vi "Facade.vi"(0 "Data In":T9, 2 "Display State In":T4={"Z_Source"={"connect"=FALSE, "Z_Source"=enum."initialize", "Z_State_heating"=enum."on"}, "Write"=FALSE, "Z1_ind"=0, "button state"=enum."init", "reset_timer"=FALSE, "load_timer"=FALSE, "end_timer"=TRUE}, 3 "Container State":T8) -> (6 "Data Out":T9, 7 "Display State Out":T4={"Z_Source"={"connect"=FALSE, "Z_Source"=enum."initialize", "Z_State_heating"=enum."on"}, "Write"=FALSE, "Z1_ind"=0, "button state"=enum."init", "reset_timer"=FALSE, "load_timer"=FALSE, "end_timer"=TRUE}, 8 "Action":T3)   [LabVIEW 2019, in "Heating.lvlib" / "Z_OnSwitch.xctl"]
uses:
  Z_OnSwitch.xctl
  Data.ctl
  <vilib>/_xctls/Container State.ctl
  State.ctl
  Z_source.ctl
  Z_State.ctl
  On_ButtonState.ctl
  <vilib>/_xctls/Action.ctl
  Z_OnSwitch.ctl
  Z_OnInd.ctl
  <vilib>/_xctls/XControlSupport.lvlib
  Timer Delay/Timers.lvlib
  Heating.lvlib
panel:
  in  "Z_OnSwitch":T1
  out "Z1 ind":T2
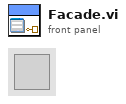
[diagram p1: front panel]
types:
  T1 = typedef "Heating.lvlib/Z_OnSwitch.xctl/Z_OnSwitch.ctl" = bool
  T2 = typedef "Heating.lvlib/Z_OnSwitch.xctl/Z_OnInd.ctl" = u8
  T3 = typedef "XControlSupport.lvlib/Action.ctl" = cluster{"Data Changed?":bool, "State Changed?":bool, "Action Name":string}
  T4 = typedef "Heating.lvlib/Z_OnSwitch.xctl/State.ctl" = cluster{"Z_Source":cluster{"connect":bool, "Z_Source":T5, "Z_State_heating":T6}, "Write":bool, "Z1_ind":u8, "button state":T7, "reset_timer":bool, "load_timer":bool, "end_timer":bool}
  T5 = typedef "Heating.lvlib/Z_source.ctl" = enum8{"initialize", "local disabled", "local hand", "hand", "auto", "dist"}
  T6 = typedef "Heating.lvlib/Z_State.ctl" = enum8{"initialization", "alarm", "disabled", "not ready", "stop ready", "reserv", "switched off", "reserv2", "switched on", "check", "on min", "decrease out", "on", "increase out", "on max"}
  T7 = typedef "Heating.lvlib/Z_OnSwitch.xctl/On_ButtonState.ctl" = enum16{"init", "not connect", "local disabled", "local hand", "switch off", "off", "switch on", "on", "auto", "dist"}
  T8 = typedef "XControlSupport.lvlib/Container State.ctl" = cluster{"Indicator?":bool, "Run Mode?":bool, " Refnum":refnum<vi>}
  T9 = typedef "Heating.lvlib/Z_OnSwitch.xctl/Data.ctl" = bool
  T10 = enum8{"Enabled", "Disabled", "Disabled and Grayed Out"}
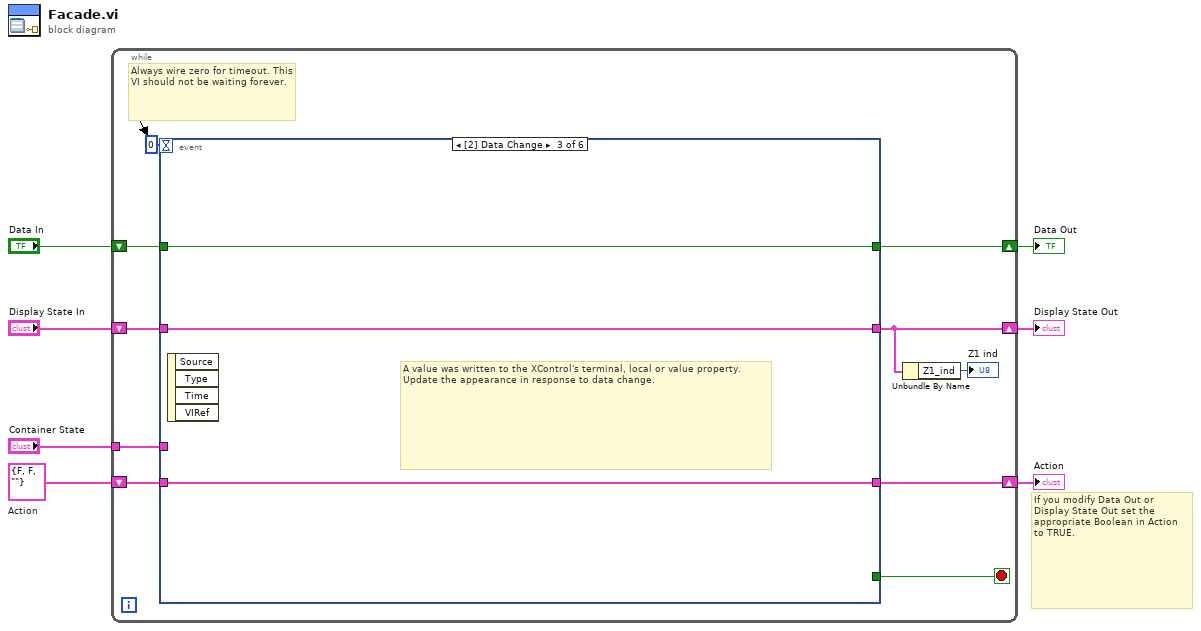
[diagram p0: block diagram]
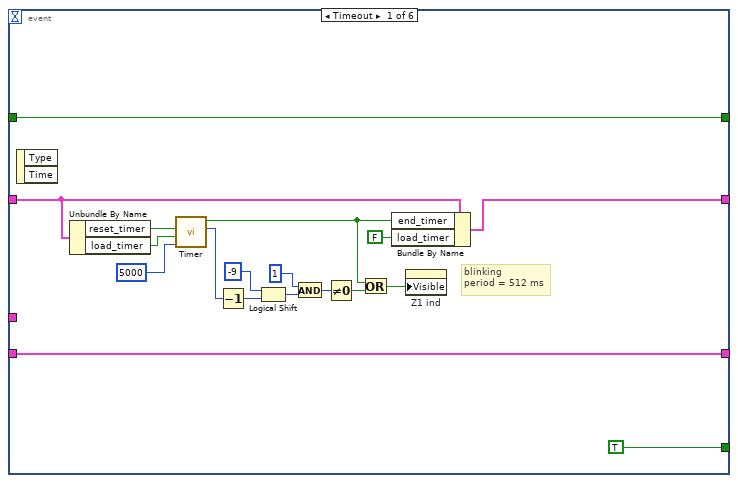
[diagram p2: hidden frame]
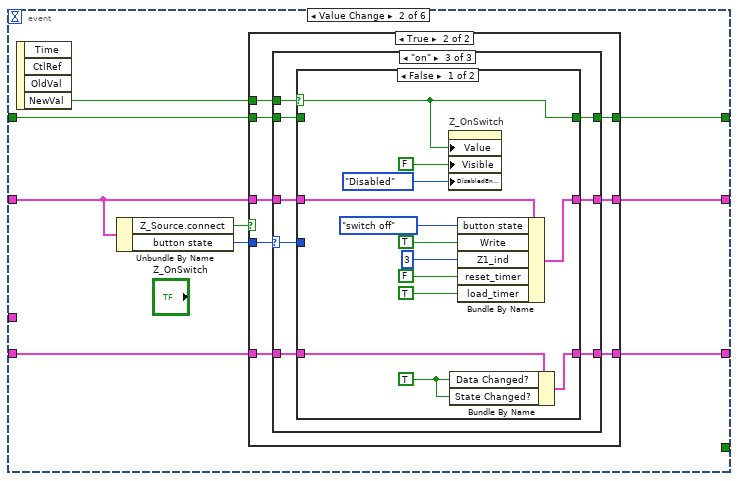
[diagram p3: hidden frame]
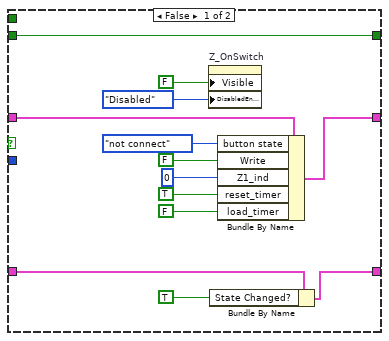
[diagram p4: hidden frame]
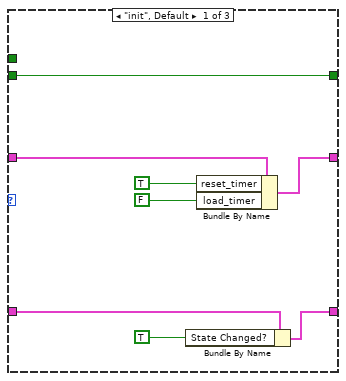
[diagram p5: hidden frame]
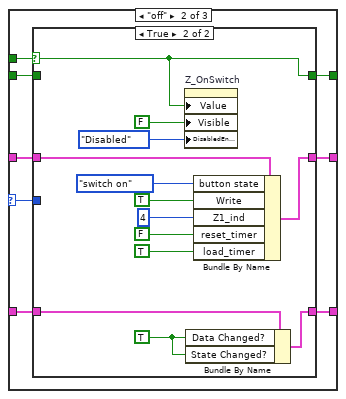
[diagram p6: hidden frame]
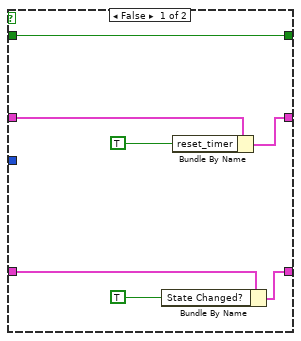
[diagram p7: hidden frame]
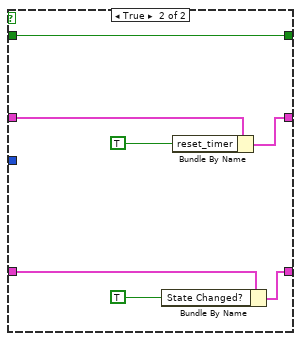
[diagram p8: hidden frame]
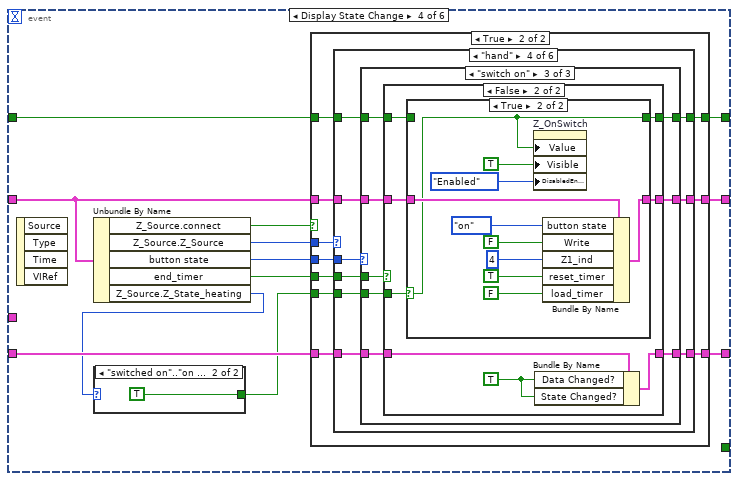
[diagram p9: hidden frame]
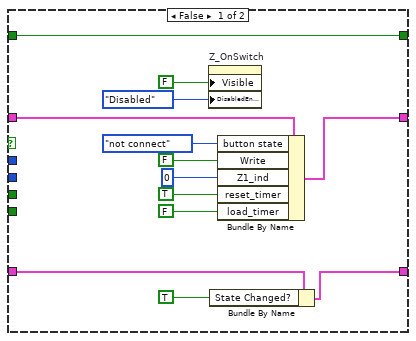
[diagram p11: hidden frame]
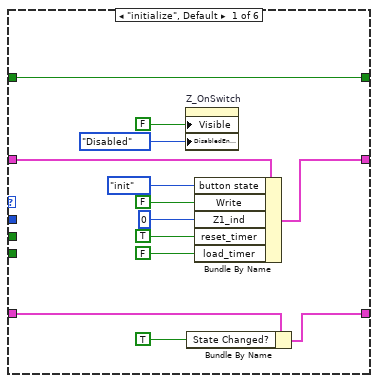
[diagram p12: hidden frame]
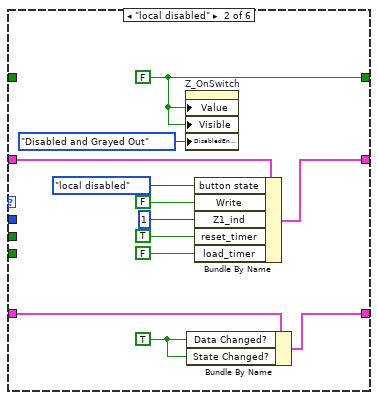
[diagram p13: hidden frame]
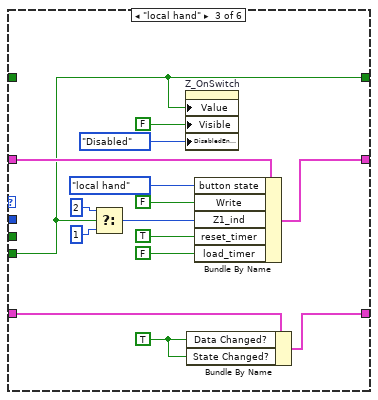
[diagram p14: hidden frame]
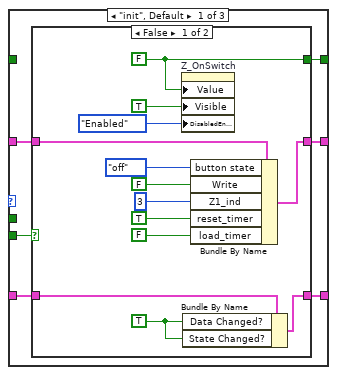
[diagram p15: hidden frame]
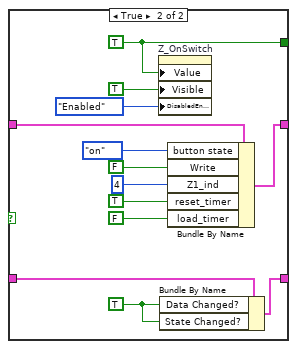
[diagram p16: hidden frame]
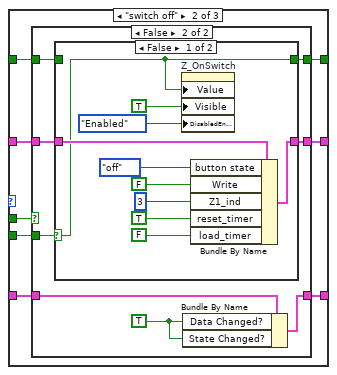
[diagram p17: hidden frame]
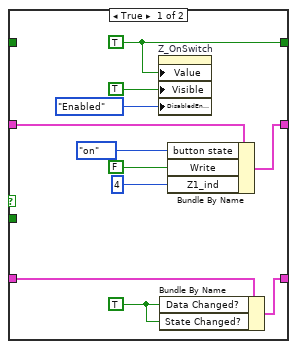
[diagram p18: hidden frame]
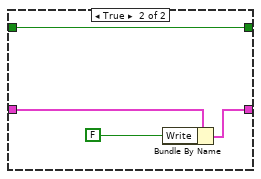
[diagram p19: hidden frame]
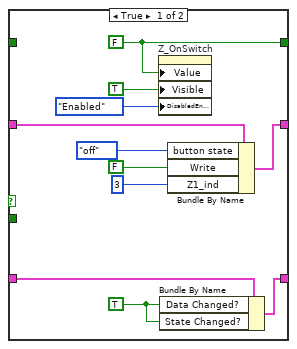
[diagram p20: hidden frame]
diagram:
  w1 = T3 {"Data Changed?"=FALSE, "State Changed?"=FALSE, "Action Name"=""}  # Action
  # "If you modify Data Out or\nDisplay State Out set the\nappropriate Boolean in Action\nto TRUE."
  n1 = while {
    shift-right: [w8] -> w4
    shift-left: "Display State In" -> [w17]
    tunnel: "Container State" -> [w14]
    shift-right: [w12] -> w7
    shift-left: "Data In" -> [w13]
    shift-right: [w10] -> w2
    shift-left: w1 -> [w11]
    stop <- w16 stop-if-true
    # "Always wire zero for timeout. This\nVI should not be waiting forever."
    n2 = event shown="[2] Data Change" {
      selector: _ -> [_ _ _ _ _ _]
      dyn-events: _ -> [_ _ _ _ _ _]
      timeout: 0 -> [_ _ _ _ _ _]
      tunnel: w17 -> [w30 w38 w131 w138 w362 w366]
      tunnel: [w29 w43 w131 w142 w362 w366] -> w8
      tunnel: [TRUE _ _ _ _ _] -> w16
      tunnel: w14 -> [_ _ _ _ w363 w367]
      tunnel: w13 -> [w33 w42 w132 w144 w361 w365]
      tunnel: [w33 w41 w132 w143 w361 w365] -> w12
      tunnel: [w34 w39 w130 w140 w360 w364] -> w10
      tunnel: w11 -> [w34 w40 w130 w141 w360 w364]
      event Timeout {
        # "blinking\nperiod = 512 ms"
        n3 = event-data() -> ()  [unwired: 1 in, 2 out]
        n4 = Unbundle By Name(w30) -> ("reset_timer"=w32:bool, "load_timer"=w31:bool)
        n5 = call "Timer.vi"("ms"=5000, "Load (F)"=w31, "Reset (F)"=w32) -> ("t ms"=w27:u32, "End"=w23:bool)  [unwired: 6 in]
        n6 = Decrement(x=w27) -> (x-1=w22:u32)
        n7 = Logical Shift(y=i16 -9, x=w22) -> (x << y=w20:u32)
        n8 = And(x=u32 1 ("y"), y=w20) -> (x .and. y?=w18:u32)
        n9 = Not Equal To 0?(x=w18) -> (x != 0?=w24:bool)
        n10 = Or(x=w23, y=w24) -> (x .or. y?=w25:bool)
        n11 = Bundle By Name(cluster=w30, "end_timer"=w23, "load_timer"=FALSE) -> (w29:T4)
        n12 = property on="Z1 ind" class="Ring (strict)"("Visible"=w25) -> ()  [unwired: 2 in, 2 out]
      }
      event Value Change {
        n13 = event-data() -> ("NewVal"=w44:T1)  [unwired: 1 in, 3 out]
        n14 = Unbundle By Name(w38) -> ("Z_Source.connect"=w37:bool, "button state"=w36:T7)
        n15 = case shown="True" w37 {
          tunnel: w36 -> [_ w65]
          tunnel: w44 -> [_ w64]
          tunnel: w38 -> [w52 w63]
          tunnel: [w51 w62] -> w43
          tunnel: w42 -> [w57 w61]
          tunnel: [w57 w60] -> w41
          tunnel: w40 -> [w49 w58]
          tunnel: [w48 w59] -> w39
          frame False {
            n16 = property on="Z_OnSwitch" class="Bool (strict)"("Visible"=FALSE ("Z_ASwitch"), "DisabledEnum"=T10."Disabled" ("Disabled")) -> ()  [unwired: 2 in, 2 out]
            n17 = Bundle By Name(cluster=w49, "State Changed?"=TRUE ("Data Changed?")) -> (w48:T3)
            n18 = Bundle By Name(cluster=w52, "button state"=On_ButtonState."not connect" ("f 3"), "Write"=FALSE ("Z_ASwitch"), "Z1_ind"=u8 0 ("Z1_ind visu"), "reset_timer"=TRUE ("Z_ASwitch"), "load_timer"=FALSE ("Z_ASwitch")) -> (w51:T4)
          }
          frame True {
            n19 = case shown="\"on\"" w65 {
              selector: w65 -> [_ w80 w108]
              tunnel: w64 -> [_ w81 w109]
              tunnel: w63 -> [w72 w79 w107]
              tunnel: [w71 w78 w106] -> w62
              tunnel: w61 -> [w70 w76 w105]
              tunnel: [w70 w77 w104] -> w60
              tunnel: [w67 w74 w102] -> w59
              tunnel: w58 -> [w68 w75 w103]
              frame "init", Default {
                # "local hand"
                n20 = Bundle By Name(cluster=w68, "State Changed?"=TRUE ("Data Changed?")) -> (w67:T3)
                n21 = Bundle By Name(cluster=w72, "reset_timer"=TRUE, "load_timer"=FALSE) -> (w71:T4)
              }
              frame "off" {
                # "local hand"
                n22 = case shown="True" w81 {
                  selector: w81 -> [_ w93]
                  tunnel: w80 -> [_ _]
                  tunnel: w79 -> [w87 w95]
                  tunnel: [w86 w94] -> w78
                  tunnel: [w85 w93] -> w77
                  tunnel: w76 -> [w85 _]
                  tunnel: w75 -> [w83 w91]
                  tunnel: [w82 w90] -> w74
                  frame False {
                    n23 = Bundle By Name(cluster=w83, "State Changed?"=TRUE ("Data Changed?")) -> (w82:T3)
                    n24 = Bundle By Name(cluster=w87, "reset_timer"=TRUE) -> (w86:T4)
                  }
                  frame True {
                    w92 = TRUE ("Data Changed?")
                    n25 = property on="Z_OnSwitch" class="Bool (strict)"("Value"=w93, "Visible"=FALSE ("Z_ASwitch"), "DisabledEnum"=T10."Disabled" ("Disabled")) -> ()  [unwired: 2 in, 2 out]
                    n26 = Bundle By Name(cluster=w91, "Data Changed?"=w92, "State Changed?"=w92) -> (w90:T3)
                    n27 = Bundle By Name(cluster=w95, "button state"=On_ButtonState."switch on" ("f 3"), "Write"=TRUE ("Z_ASwitch"), "Z1_ind"=u8 4 ("Z1_ind visu"), "reset_timer"=FALSE ("Z_ASwitch"), "load_timer"=TRUE ("Z_ASwitch")) -> (w94:T4)
                  }
                }
              }
              frame "on" {
                # "local hand"
                n28 = case shown="False" w109 {
                  selector: w109 -> [w114 _]
                  tunnel: w108 -> [_ _]
                  tunnel: w107 -> [w116 w128]
                  tunnel: [w115 w127] -> w106
                  tunnel: w105 -> [_ w129]
                  tunnel: [w114 w129] -> w104
                  tunnel: w103 -> [w112 w124]
                  tunnel: [w111 w123] -> w102
                  frame False {
                    w113 = TRUE ("Data Changed?")
                    n29 = property on="Z_OnSwitch" class="Bool (strict)"("Value"=w114, "Visible"=FALSE ("Z_ASwitch"), "DisabledEnum"=T10."Disabled" ("Disabled")) -> ()  [unwired: 2 in, 2 out]
                    n30 = Bundle By Name(cluster=w112, "Data Changed?"=w113, "State Changed?"=w113) -> (w111:T3)
                    n31 = Bundle By Name(cluster=w116, "button state"=On_ButtonState."switch off" ("f 3"), "Write"=TRUE ("Z_ASwitch"), "Z1_ind"=u8 3 ("Z1_ind visu"), "reset_timer"=FALSE ("Z_ASwitch"), "load_timer"=TRUE ("Z_ASwitch")) -> (w115:T4)
                  }
                  frame True {
                    n32 = Bundle By Name(cluster=w124, "State Changed?"=TRUE ("Data Changed?")) -> (w123:T3)
                    n33 = Bundle By Name(cluster=w128, "reset_timer"=TRUE ("Z1_ind_blinking")) -> (w127:T4)
                  }
                }
              }
            }
          }
        }
      }
      event Data Change {
        # "A value was written to the XControl's terminal, local or value property.\nUpdate the appearance in response to data change."
        n34 = event-data() -> ()  [unwired: 1 in, 4 out]
      }
      event Display State Change {
        n35 = event-data() -> ()  [unwired: 1 in, 4 out]
        n36 = Unbundle By Name(w138) -> ("Z_Source.connect"=w139:bool, "Z_Source.Z_Source"=w136:T5, "button state"=w135:T7, "end_timer"=w137:bool, "Z_Source.Z_State_heating"=w134:T6)
        n37 = case shown="\"switched on\"..\"on max\"" w134 {
          tunnel: [_ TRUE] -> w133
          frame "initialization", Default {
          }
          frame "switched on".."on max" {
          }
        }
        n38 = case shown="True" w139 {
          tunnel: w136 -> [_ w168]
          tunnel: w138 -> [w153 w167]
          tunnel: [w152 w166] -> w142
          tunnel: w144 -> [w158 w165]
          tunnel: [w158 w164] -> w143
          tunnel: w141 -> [w150 w162]
          tunnel: [w149 w163] -> w140
          tunnel: w137 -> [_ w161]
          tunnel: w135 -> [_ w160]
          tunnel: w133 -> [_ w159]
          frame False {
            n39 = property on="Z_OnSwitch" class="Bool (strict)"("Visible"=FALSE ("Z_ASwitch"), "DisabledEnum"=T10."Disabled" ("Disabled")) -> ()  [unwired: 2 in, 2 out]
            n40 = Bundle By Name(cluster=w150, "State Changed?"=TRUE ("Data Changed?")) -> (w149:T3)
            n41 = Bundle By Name(cluster=w153, "button state"=On_ButtonState."not connect" ("f 3"), "Write"=FALSE ("Z_ASwitch"), "Z1_ind"=u8 0 ("Z1_ind visu"), "reset_timer"=TRUE ("Z_ASwitch"), "load_timer"=FALSE ("Z_ASwitch")) -> (w152:T4)
          }
          frame True {
            n42 = case shown="\"hand\"" w168 {
              tunnel: w167 -> [w181 w193 w208 w214 w346 w359]
              tunnel: [w180 w192 w207 w216 w345 w358] -> w166
              tunnel: w165 -> [w170 _ _ w215 _ _]
              tunnel: [w170 w183 w194 w217 w332 w347] -> w164
              tunnel: [w178 w190 w205 w210 w343 w356] -> w163
              tunnel: w162 -> [w179 w191 w206 w211 w344 w357]
              tunnel: w161 -> [_ _ _ w213 _ _]
              tunnel: w160 -> [_ _ _ w212 _ _]
              tunnel: w159 -> [_ _ w194 w209 w332 w347]
              frame "initialize", Default {
                # "local hand"
                n43 = property on="Z_OnSwitch" class="Bool (strict)"("Visible"=FALSE ("Z_ASwitch"), "DisabledEnum"=T10."Disabled" ("Disabled")) -> ()  [unwired: 2 in, 2 out]
                n44 = Bundle By Name(cluster=w179, "State Changed?"=TRUE ("Data Changed?")) -> (w178:T3)
                n45 = Bundle By Name(cluster=w181, "button state"=On_ButtonState."init" ("f 3"), "Write"=FALSE ("Z_ASwitch"), "Z1_ind"=u8 0 ("Z1_ind visu"), "reset_timer"=TRUE ("Z_ASwitch"), "load_timer"=FALSE ("Z_ASwitch")) -> (w180:T4)
              }
              frame "local disabled" {
                w182 = TRUE ("Data Changed?")
                w183 = FALSE ("Z_ASwitch")
                # "local hand"
                n46 = property on="Z_OnSwitch" class="Bool (strict)"("Value"=w183, "Visible"=w183, "DisabledEnum"=T10."Disabled and Grayed Out" ("Disabled")) -> ()  [unwired: 2 in, 2 out]
                n47 = Bundle By Name(cluster=w191, "Data Changed?"=w182, "State Changed?"=w182) -> (w190:T3)
                n48 = Bundle By Name(cluster=w193, "button state"=On_ButtonState."local disabled" ("f 3"), "Write"=FALSE ("Z_ASwitch"), "Z1_ind"=u8 1 ("Z1_ind visu"), "reset_timer"=TRUE ("Z_ASwitch"), "load_timer"=FALSE ("Z_ASwitch")) -> (w192:T4)
              }
              frame "local hand" {
                w198 = TRUE ("Data Changed?")
                # "local hand"
                n49 = Select(t=u8 2 ("Z1_ind visu"), s=w194, f=u8 1 ("Z1_ind visu")) -> (s? t:f=w195:u8)
                n50 = property on="Z_OnSwitch" class="Bool (strict)"("Value"=w194, "Visible"=FALSE ("Z_ASwitch"), "DisabledEnum"=T10."Disabled" ("Disabled")) -> ()  [unwired: 2 in, 2 out]
                n51 = Bundle By Name(cluster=w206, "Data Changed?"=w198, "State Changed?"=w198) -> (w205:T3)
                n52 = Bundle By Name(cluster=w208, "button state"=On_ButtonState."local hand" ("f 3"), "Write"=FALSE ("Z_ASwitch"), "Z1_ind"=w195, "reset_timer"=TRUE ("Z_ASwitch"), "load_timer"=FALSE ("Z_ASwitch")) -> (w207:T4)
              }
              frame "hand" {
                # "local hand"
                n53 = case shown="\"switch on\"" w212 {
                  tunnel: w213 -> [_ w257 w298]
                  tunnel: w214 -> [w223 w251 w292]
                  tunnel: [w219 w252 w293] -> w216
                  tunnel: w215 -> [_ w256 w297]
                  tunnel: [w220 w255 w296] -> w217
                  tunnel: w211 -> [w222 w253 w294]
                  tunnel: [w221 w254 w295] -> w210
                  tunnel: w209 -> [w218 w250 w291]
                  frame "init", Default {
                    n54 = case shown="False" w218 {
                      tunnel: w223 -> [w233 w246]
                      tunnel: w222 -> [w231 w244]
                      tunnel: [w230 w243] -> w221
                      tunnel: [w229 w242] -> w220
                      tunnel: [w224 w237] -> w219
                      frame False {
                        w225 = TRUE ("Data Changed?")
                        w229 = FALSE ("Z_ASwitch")
                        n55 = property on="Z_OnSwitch" class="Bool (strict)"("Value"=w229, "Visible"=TRUE ("Z_ASwitch"), "DisabledEnum"=T10."Enabled" ("Disabled")) -> ()  [unwired: 2 in, 2 out]
                        n56 = Bundle By Name(cluster=w231, "Data Changed?"=w225, "State Changed?"=w225) -> (w230:T3)
                        n57 = Bundle By Name(cluster=w233, "button state"=On_ButtonState."off" ("f 3"), "Write"=FALSE ("Z_ASwitch"), "Z1_ind"=u8 3 ("Z1_ind visu"), "reset_timer"=TRUE ("Z_ASwitch"), "load_timer"=FALSE ("Z_ASwitch")) -> (w224:T4)
                      }
                      frame True {
                        w238 = TRUE ("Data Changed?")
                        w242 = TRUE ("Z_ASwitch")
                        n58 = property on="Z_OnSwitch" class="Bool (strict)"("Value"=w242, "Visible"=TRUE ("Z_ASwitch"), "DisabledEnum"=T10."Enabled" ("Disabled")) -> ()  [unwired: 2 in, 2 out]
                        n59 = Bundle By Name(cluster=w244, "Data Changed?"=w238, "State Changed?"=w238) -> (w243:T3)
                        n60 = Bundle By Name(cluster=w246, "button state"=On_ButtonState."on" ("f 3"), "Write"=FALSE ("Z_ASwitch"), "Z1_ind"=u8 4 ("Z1_ind visu"), "reset_timer"=TRUE ("Z_ASwitch"), "load_timer"=FALSE ("Z_ASwitch")) -> (w237:T4)
                      }
                    }
                  }
                  frame "switch off" {
                    n61 = case shown="False" w257 {
                      tunnel: w251 -> [w268 w276]
                      tunnel: [w267 w275] -> w252
                      tunnel: w256 -> [_ w269]
                      tunnel: [w260 w271] -> w255
                      tunnel: [w265 w273] -> w254
                      tunnel: w253 -> [w266 w274]
                      tunnel: w250 -> [_ w270]
                      frame True {
                        w262 = TRUE ("Data Changed?")
                        w260 = TRUE ("Z_ASwitch")
                        # "local hand"
                        n62 = property on="Z_OnSwitch" class="Bool (strict)"("Value"=w260, "Visible"=TRUE ("Z_ASwitch"), "DisabledEnum"=T10."Enabled" ("Disabled")) -> ()  [unwired: 2 in, 2 out]
                        n63 = Bundle By Name(cluster=w266, "Data Changed?"=w262, "State Changed?"=w262) -> (w265:T3)
                        n64 = Bundle By Name(cluster=w268, "button state"=On_ButtonState."on" ("f 3"), "Write"=FALSE ("Z_ASwitch"), "Z1_ind"=u8 4 ("Z1_ind visu")) -> (w267:T4)
                      }
                      frame False {
                        w272 = TRUE ("Data Changed?")
                        # "local hand"
                        n65 = case shown="False" w270 {
                          selector: w270 -> [w277 _]
                          tunnel: w276 -> [w286 w287]
                          tunnel: [w285 w288] -> w275
                          tunnel: [w277 w290] -> w271
                          tunnel: w269 -> [_ w290]
                          frame False {
                            n66 = property on="Z_OnSwitch" class="Bool (strict)"("Value"=w277, "Visible"=TRUE ("Z_ASwitch"), "DisabledEnum"=T10."Enabled" ("Disabled")) -> ()  [unwired: 2 in, 2 out]
                            n67 = Bundle By Name(cluster=w286, "button state"=On_ButtonState."off" ("f 3"), "Write"=FALSE ("Z_ASwitch"), "Z1_ind"=u8 3 ("Z1_ind visu"), "reset_timer"=TRUE ("Z_ASwitch"), "load_timer"=FALSE ("Z_ASwitch")) -> (w285:T4)
                          }
                          frame True {
                            n68 = Bundle By Name(cluster=w287, "Write"=FALSE ("Z_ASwitch")) -> (w288:T4)
                          }
                        }
                        n69 = Bundle By Name(cluster=w274, "Data Changed?"=w272, "State Changed?"=w272) -> (w273:T3)
                      }
                    }
                  }
                  frame "switch on" {
                    n70 = case shown="False" w298 {
                      tunnel: w292 -> [w309 w317]
                      tunnel: [w308 w316] -> w293
                      tunnel: w297 -> [_ w310]
                      tunnel: [w301 w312] -> w296
                      tunnel: [w306 w314] -> w295
                      tunnel: w294 -> [w307 w315]
                      tunnel: w291 -> [_ w311]
                      frame True {
                        w303 = TRUE ("Data Changed?")
                        w301 = FALSE ("Z_ASwitch")
                        # "local hand"
                        n71 = property on="Z_OnSwitch" class="Bool (strict)"("Value"=w301, "Visible"=TRUE ("Z_ASwitch"), "DisabledEnum"=T10."Enabled" ("Disabled")) -> ()  [unwired: 2 in, 2 out]
                        n72 = Bundle By Name(cluster=w307, "Data Changed?"=w303, "State Changed?"=w303) -> (w306:T3)
                        n73 = Bundle By Name(cluster=w309, "button state"=On_ButtonState."off" ("f 3"), "Write"=FALSE ("Z_ASwitch"), "Z1_ind"=u8 3 ("Z1_ind visu")) -> (w308:T4)
                      }
                      frame False {
                        w313 = TRUE ("Data Changed?")
                        # "local hand"
                        n74 = case shown="True" w311 {
                          selector: w311 -> [_ w322]
                          tunnel: w317 -> [w318 w331]
                          tunnel: [w319 w330] -> w316
                          tunnel: [w321 w322] -> w312
                          tunnel: w310 -> [w321 _]
                          frame False {
                            n75 = Bundle By Name(cluster=w318, "Write"=FALSE ("Z_ASwitch")) -> (w319:T4)
                          }
                          frame True {
                            n76 = property on="Z_OnSwitch" class="Bool (strict)"("Value"=w322, "Visible"=TRUE ("Z_ASwitch"), "DisabledEnum"=T10."Enabled" ("Disabled")) -> ()  [unwired: 2 in, 2 out]
                            n77 = Bundle By Name(cluster=w331, "button state"=On_ButtonState."on" ("f 3"), "Write"=FALSE ("Z_ASwitch"), "Z1_ind"=u8 4 ("Z1_ind visu"), "reset_timer"=TRUE ("Z_ASwitch"), "load_timer"=FALSE ("Z_ASwitch")) -> (w330:T4)
                          }
                        }
                        n78 = Bundle By Name(cluster=w315, "Data Changed?"=w313, "State Changed?"=w313) -> (w314:T3)
                      }
                    }
                  }
                }
              }
              frame "auto" {
                w336 = TRUE ("Data Changed?")
                # "local hand"
                n79 = Select(t=u8 4 ("Z1_ind visu"), s=w332, f=u8 3 ("Z1_ind visu")) -> (s? t:f=w333:u8)
                n80 = property on="Z_OnSwitch" class="Bool (strict)"("Value"=w332, "Visible"=FALSE ("Z_ASwitch"), "DisabledEnum"=T10."Disabled" ("Disabled")) -> ()  [unwired: 2 in, 2 out]
                n81 = Bundle By Name(cluster=w344, "Data Changed?"=w336, "State Changed?"=w336) -> (w343:T3)
                n82 = Bundle By Name(cluster=w346, "button state"=On_ButtonState."auto" ("f 3"), "Write"=FALSE ("Z_ASwitch"), "Z1_ind"=w333, "reset_timer"=TRUE ("Z_ASwitch"), "load_timer"=FALSE ("Z_ASwitch")) -> (w345:T4)
              }
              frame "dist" {
                w348 = TRUE ("Data Changed?")
                # "local hand"
                n83 = property on="Z_OnSwitch" class="Bool (strict)"("Value"=w347, "Visible"=FALSE ("Z_ASwitch"), "DisabledEnum"=T10."Disabled" ("Disabled")) -> ()  [unwired: 2 in, 2 out]
                n84 = Bundle By Name(cluster=w357, "Data Changed?"=w348, "State Changed?"=w348) -> (w356:T3)
                n85 = Bundle By Name(cluster=w359, "button state"=On_ButtonState."dist" ("f 3"), "Write"=FALSE ("Z_ASwitch"), "Z1_ind"=u8 5 ("Z1_ind visu"), "reset_timer"=TRUE ("Z_ASwitch"), "load_timer"=FALSE ("Z_ASwitch")) -> (w358:T4)
              }
            }
          }
        }
      }
      event Direction Change {
        # "The direction of the XControl changed from a control to an indicator or vice versa. Update the appearance accordingly."
        n86 = event-data() -> ()  [unwired: 1 in, 4 out]
        n87 = Unbundle By Name(w363) -> ()  [unwired: 1 out]
      }
      event Exec State Change {
        # "The VI owning the XControl changed from Edit Mode  to Run Mode or vice versa.\nUpdate the appearance accordingly."
        # "Handle Edit Mode & Run Mode\ncase differently"
        n88 = event-data() -> ()  [unwired: 1 in, 4 out]
        n89 = Unbundle By Name(w367) -> ()  [unwired: 1 out]
      }
    }
    n90 = Unbundle By Name(w8) -> ("Z1_ind"=→"Z1 ind":u8)
  }
  "Display State Out" <- w4
  "Data Out" <- w7
  "Action" <- w2
